vi "ixon.vi"() -> ()   [LabVIEW 2016]
uses:
  <userlib>/atmcd64d.llb/Shutter_mode typedef.ctl
  <userlib>/atmcd64d.llb/Error Code Enum typedef.ctl
  <userlib>/atmcd64d.llb/Shutter_type typedef.ctl
  <userlib>/atmcd64d.llb/FanMode_mode typedef.ctl
  <userlib>/atmcd64d.llb/ReadMode_mode typedef.ctl
  <userlib>/atmcd64d.llb/HSSpeed_type typedef.ctl
  <userlib>/atmcd64d.llb/AcquisitionMode_mode typedef.ctl
  <vilib>/Utility/miscctls.llb/LVStringsAndValuesArrayTypeDef_U16.ctl
  <vilib>/Instr/_visa.llb/VISA Configure Serial Port (Instr).vi
panel:
  in  "Tab Control":T1(tab)
  out "DLL error code from ini":u32
  out "model":string
  out "temp. status 2":T2
  out "temperature 2":i32
  in  "set temperature 2":i32
  in  "VSS (s)":u16(ring) items=["0.300000", "0.500000", "0.900000", "1.700000", "3.300000"]
  in  "HSS (MHz)":i32(ring) items=["3", "1"]
  in  "shutter":T3
  in  "exposure time (s)":sgl=0.01 step=0.001 format="%.4f"
  in  "Take shot":bool
  out "aquire status":T2
  out "Return  from Get Acquired Data":u32
  in  "live view":bool
  in  "capture stop":bool
  out "Allowed \nVertical \nShift Speed\n(seconds)":sgl[](array[numeric])
  out "Allowed \nHorizontal \nShift Speed\n(MHz)":sgl[](array[numeric])
  in  "File name":string
  in  "Path":path=path "C:/Users/Administrator/Desktop/test.tiff"
  in  "scan":bool
  in  "total scan length(mm)":dbl=25.0
  in  "distance(mm)":i32=153
  in  "lens focal length(mm)":i32=23
  out "recovering temperature":bool
  in  "Bandwidth":dbl
  in  "scan again":bool
  out "Waveform Graph":i32[](graph)
  in  "index (page) 2":i32(slide)=200 scale=0.0..512.0
  in  "Y Scale Range (mm)":dbl=67.0
  in  "stop":bool
  in  "file path (use dialog)":path=path "C:/Users/Administrator/Desktop/binary.txt"
  out "size(s) 2":i32[](array[numeric])
  out "size(s)":i32[](array[numeric])
  out "Numeric 2":i32
  out "status":T2
  out "Return  from Get Acquired Data 2":u32
  out "Intensity Graph 2":i32[][](graph)
  out "DLL error code":u32
  out "Intensity Graph":i32[][](graph)
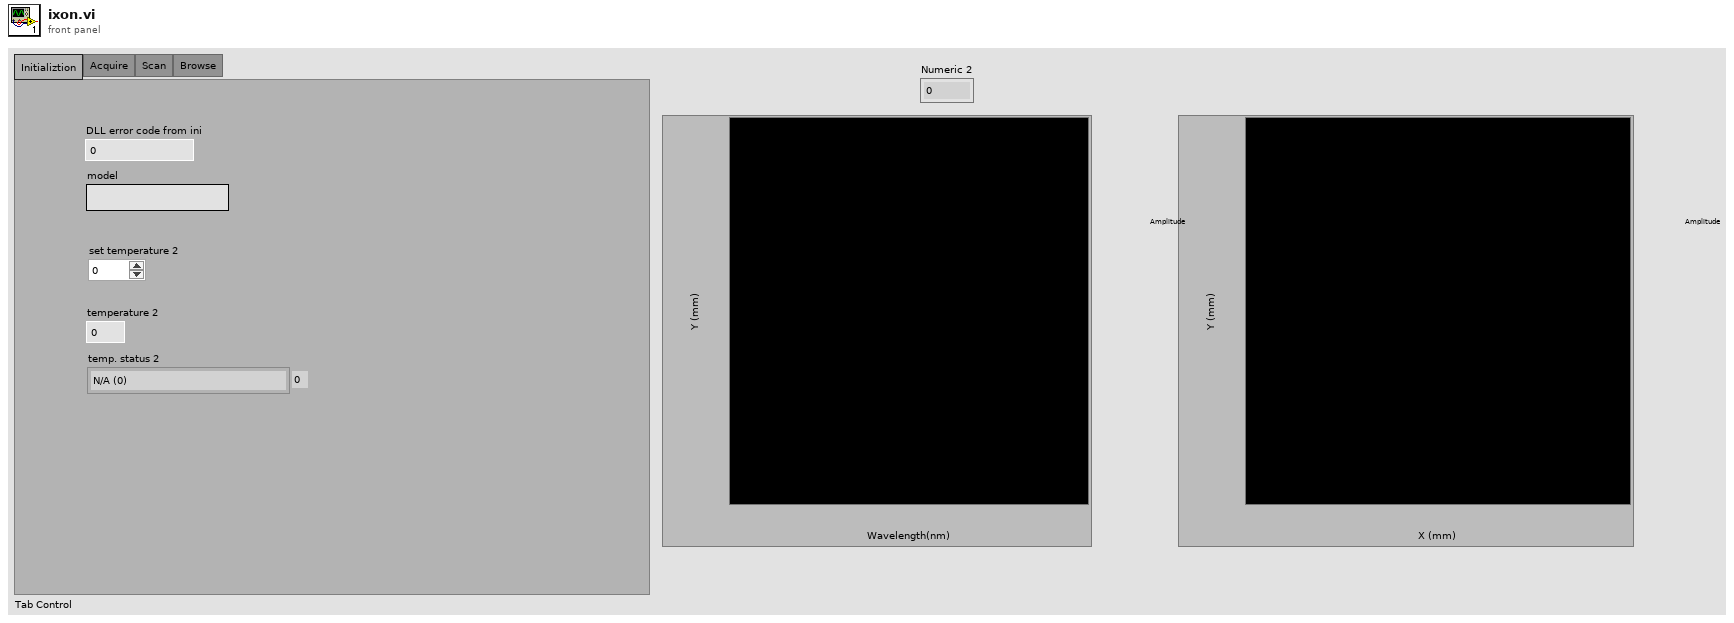
[diagram p1: front panel]
types:
  T1 = enum32{"Initializtion", "Acquire", "Scan", "Browse"}
  T2 = typedef "Error Code Enum typedef.ctl" = enum32{"N/A (0)", "DRV_ERROR_CODES", "DRV_SUCCESS", "DRV_VXDNOTINSTALLED", "DRV_ERROR_SCAN", "DRV_ERROR_CHECK_SUM", "DRV_ERROR_FILELOAD", "DRV_UNKNOWN_FUNC", "DRV_ERROR_VXD_INIT", "DRV_ERROR_ADDRESS", "DRV_ERROR_PAGELOCK", "DRV_ERROR_PAGEUNLOCK", "DRV_ERROR_BOARDTEST", "DRV_ERROR_ACK", "DRV_ERROR_UP_FIFO", "DRV_ERROR_PATTERN", "N/A (16)", "DRV_ACQUISITION_ERRORS", "DRV_ACQ_BUFFER", "DRV_ACQ_DOWNFIFO_FULL", "DRV_PROC_UNKONWN_INSTRUCTION", "DRV_ILLEGAL_OP_CODE", "DRV_KINETIC_TIME_NOT_MET", "DRV_ACCUM_TIME_NOT_MET", "DRV_NO_NEW_DATA", "N/A (25)", "DRV_SPOOLERROR", "N/A (27)", "N/A (28)", "N/A (29)", "N/A (30)", "N/A (31)", "N/A (32)", "DRV_TEMPERATURE_CODES", "DRV_TEMPERATURE_OFF", "DRV_TEMPERATURE_NOT_STABILIZED", "DRV_TEMPERATURE_STABILIZED", "DRV_TEMPERATURE_NOT_REACHED", "DRV_TEMPERATURE_OUT_RANGE", "DRV_TEMPERATURE_NOT_SUPPORTED", "DRV_TEMPERATURE_DRIFT", "N/A (41)", "N/A (42)", "N/A (43)", "N/A (44)", "N/A (45)", "N/A (46)", "N/A (47)", "N/A (48)", "DRV_GENERAL_ERRORS", "DRV_INVALID_AUX", "DRV_COF_NOTLOADED", "DRV_FPGAPROG", "DRV_FLEXERROR", "DRV_GPIBERROR", "N/A (55)", "N/A (56)", "N/A (57)", "N/A (58)", "N/A (59)", "N/A (60)", "N/A (61)", "N/A (62)", "N/A (63)", "DRV_DATATYPE", "DRV_DRIVER_ERRORS", "DRV_P1INVALID", "DRV_P2INVALID", "DRV_P3INVALID", "DRV_P4INVALID", "DRV_INIERROR", "DRV_COFERROR", "DRV_ACQUIRING", "DRV_IDLE", "DRV_TEMPCYCLE", "DRV_NOT_INITIALIZED", "DRV_P5INVALID", "DRV_P6INVALID", "DRV_INVALID_MODE", "DRV_INVALID_FILTER", "DRV_I2CERRORS", "DRV_I2CDEVNOTFOUND", "DRV_I2CTIMEOUT", "DRV_P7INVALID", "N/A (84)", "N/A (85)", "N/A (86)", "N/A (87)", "N/A (88)", "N/A (89)", "DRV_IOCERROR", "DRV_VRMVERSIONERROR"}
  T3 = typedef "Shutter_mode typedef.ctl" = enum16{"Auto", "Open", "Close", "N/A (3)", "Open FVB Series", "Open Any Series"}
  T4 = typedef "FanMode_mode typedef.ctl" = enum16{"fan on full", "fan on low", "fan off"}
  T5 = typedef "Shutter_type typedef.ctl" = enum16{"TTL Low", "TTL High"}
  T6 = typedef "LVStringsAndValuesArrayTypeDef_U16.ctl" = cluster{"String":string, "Value":u16}[]
  T7 = typedef "AcquisitionMode_mode typedef.ctl" = enum16{"Reserved (0)", "Single Scan", "Accumulate", "Kinetics", "Fast Kinetics", "Run Till Abort", "Reserved (6)", "Reserved (7)", "Reserved (8)", "Time Delayed Integration"}
  T8 = typedef "ReadMode_mode typedef.ctl" = enum16{"Full Vertical Binning", "Multi-Track", "Random-Track", "Single-Track", "Image"}
  T9 = typedef "HSSpeed_type typedef.ctl" = enum16{"EM Amp", "Conventional Amp"}
  T10 = enum16{"big-endian, network order", "native, host order", "little-endian"}
  T11 = typedef "LVPoint32TypeDef.ctl" = cluster{"Horizontal":i32, "Vertical":i32}
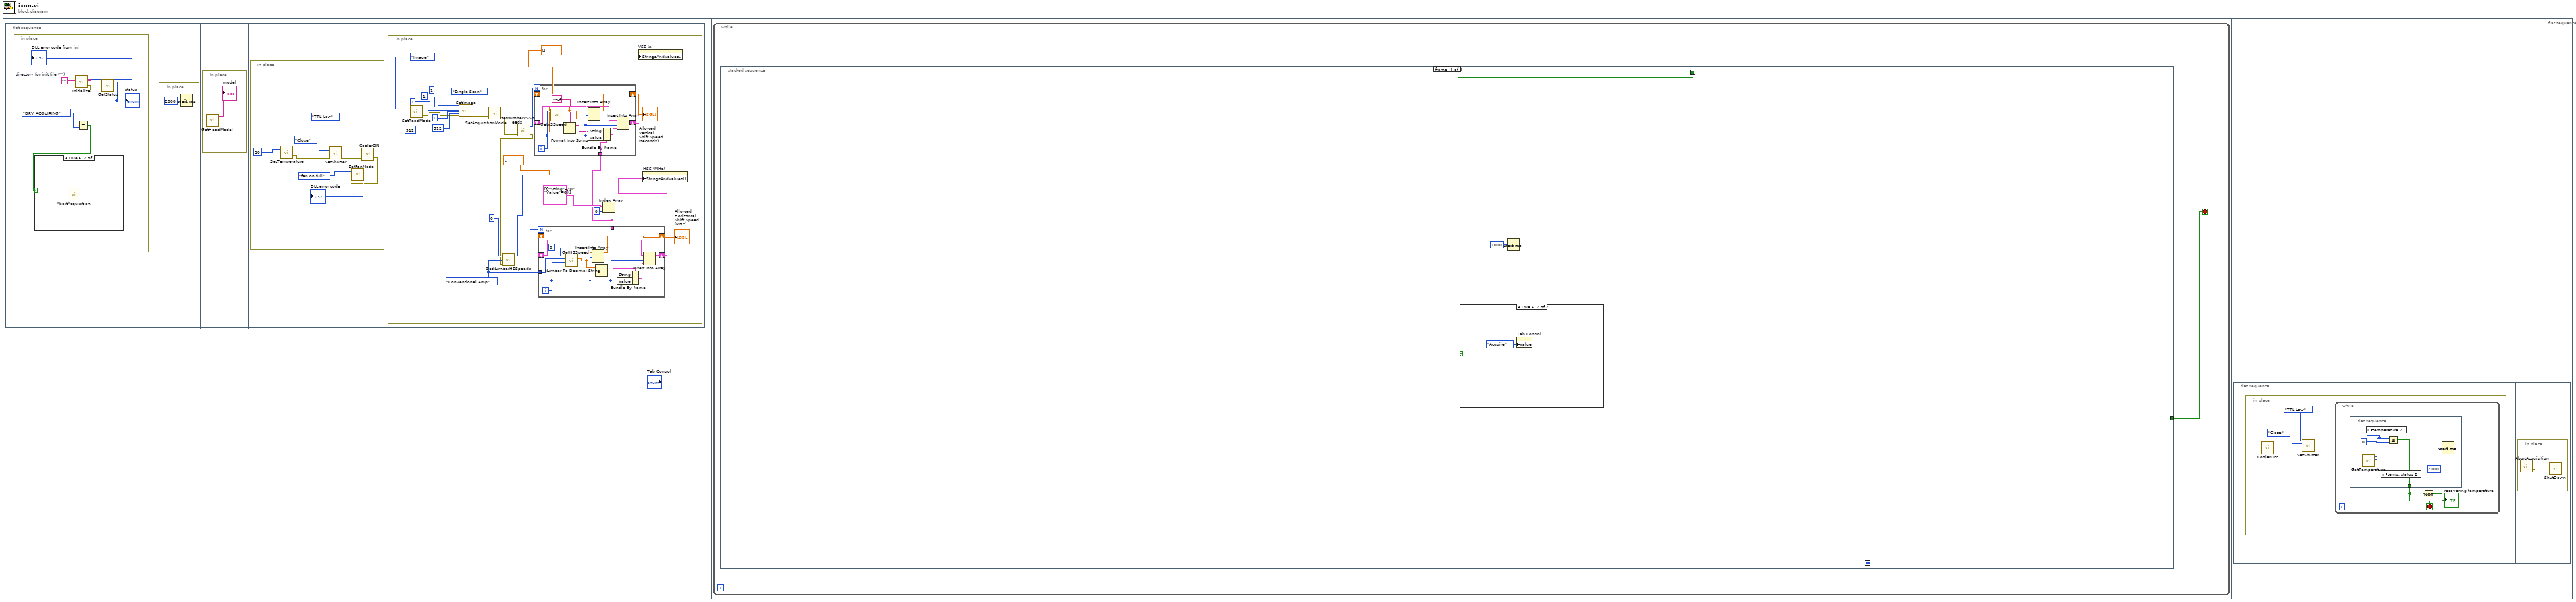
[diagram p0: block diagram]
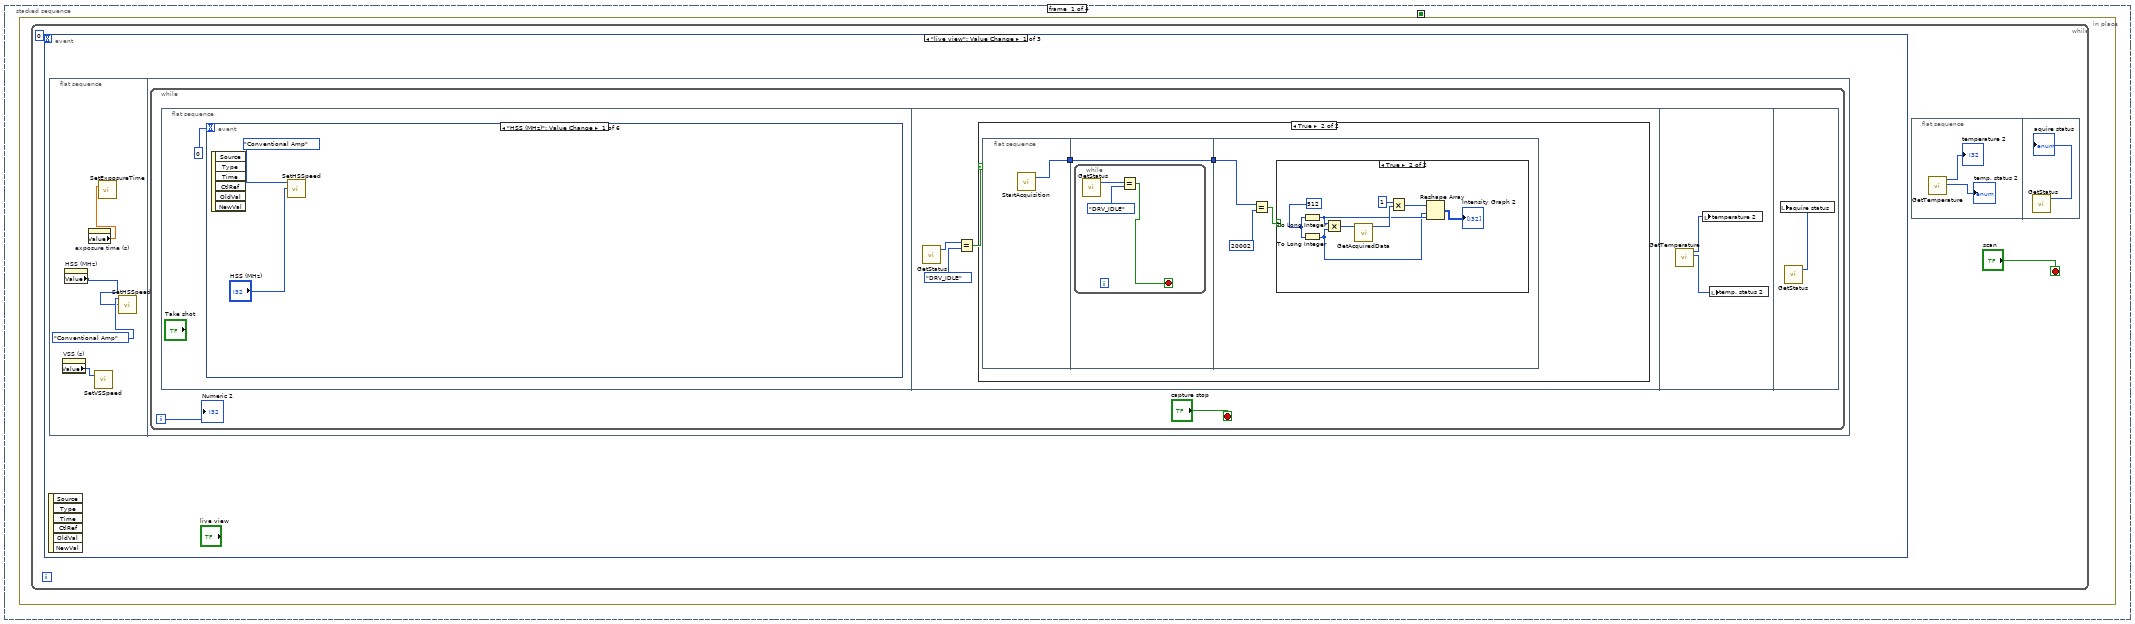
[diagram p3: hidden frame]
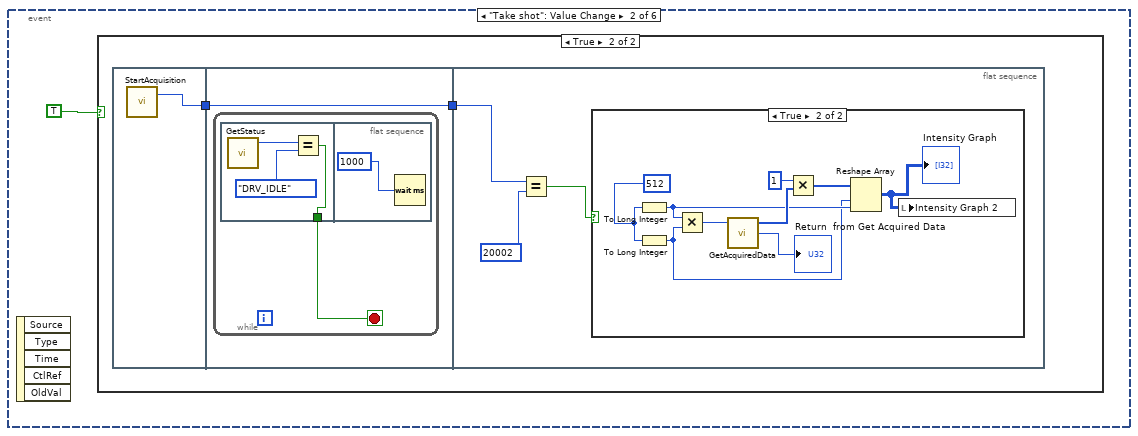
[diagram p4: hidden frame]
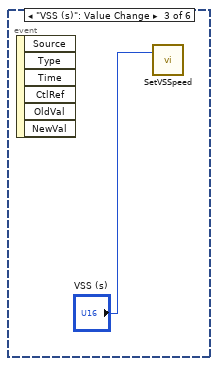
[diagram p7: hidden frame]
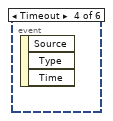
[diagram p8: hidden frame]
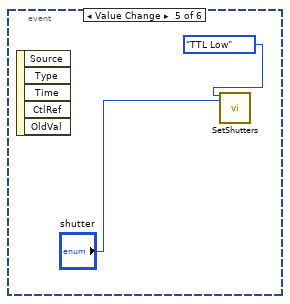
[diagram p9: hidden frame]
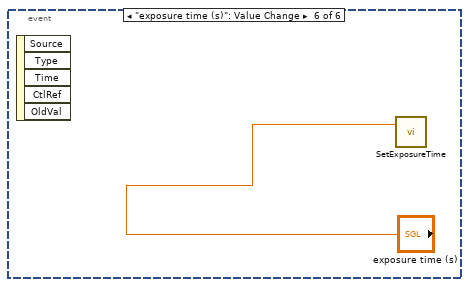
[diagram p10: hidden frame]
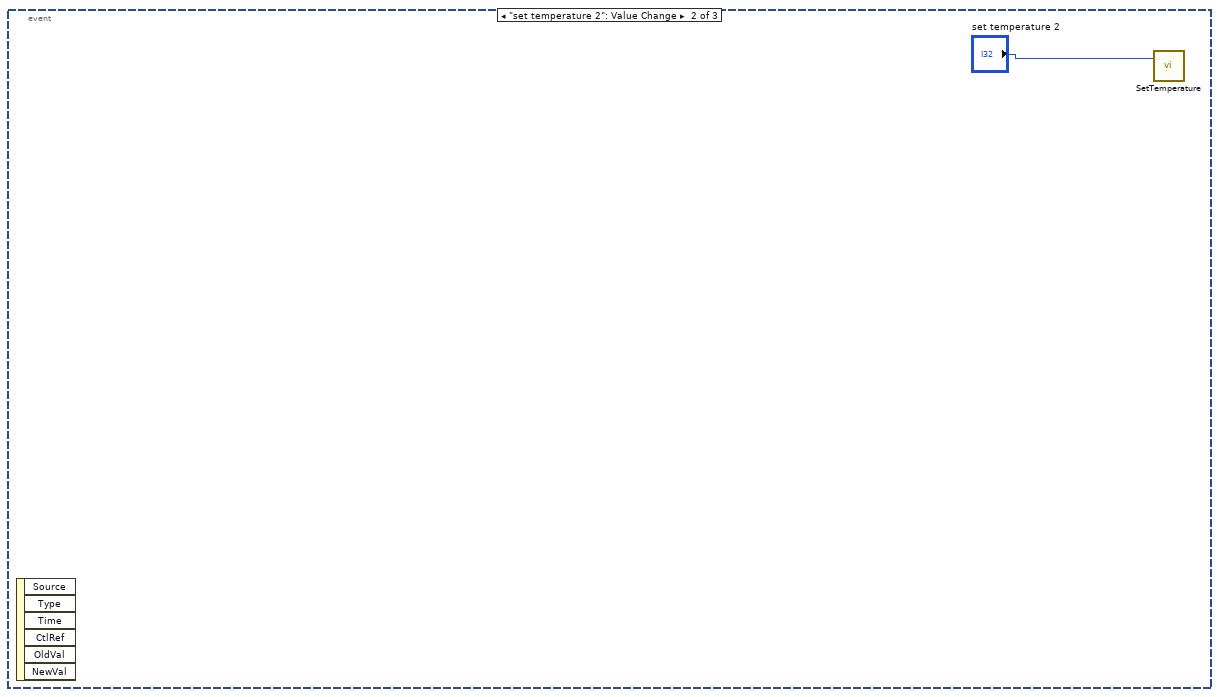
[diagram p13: hidden frame]
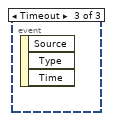
[diagram p14: hidden frame]
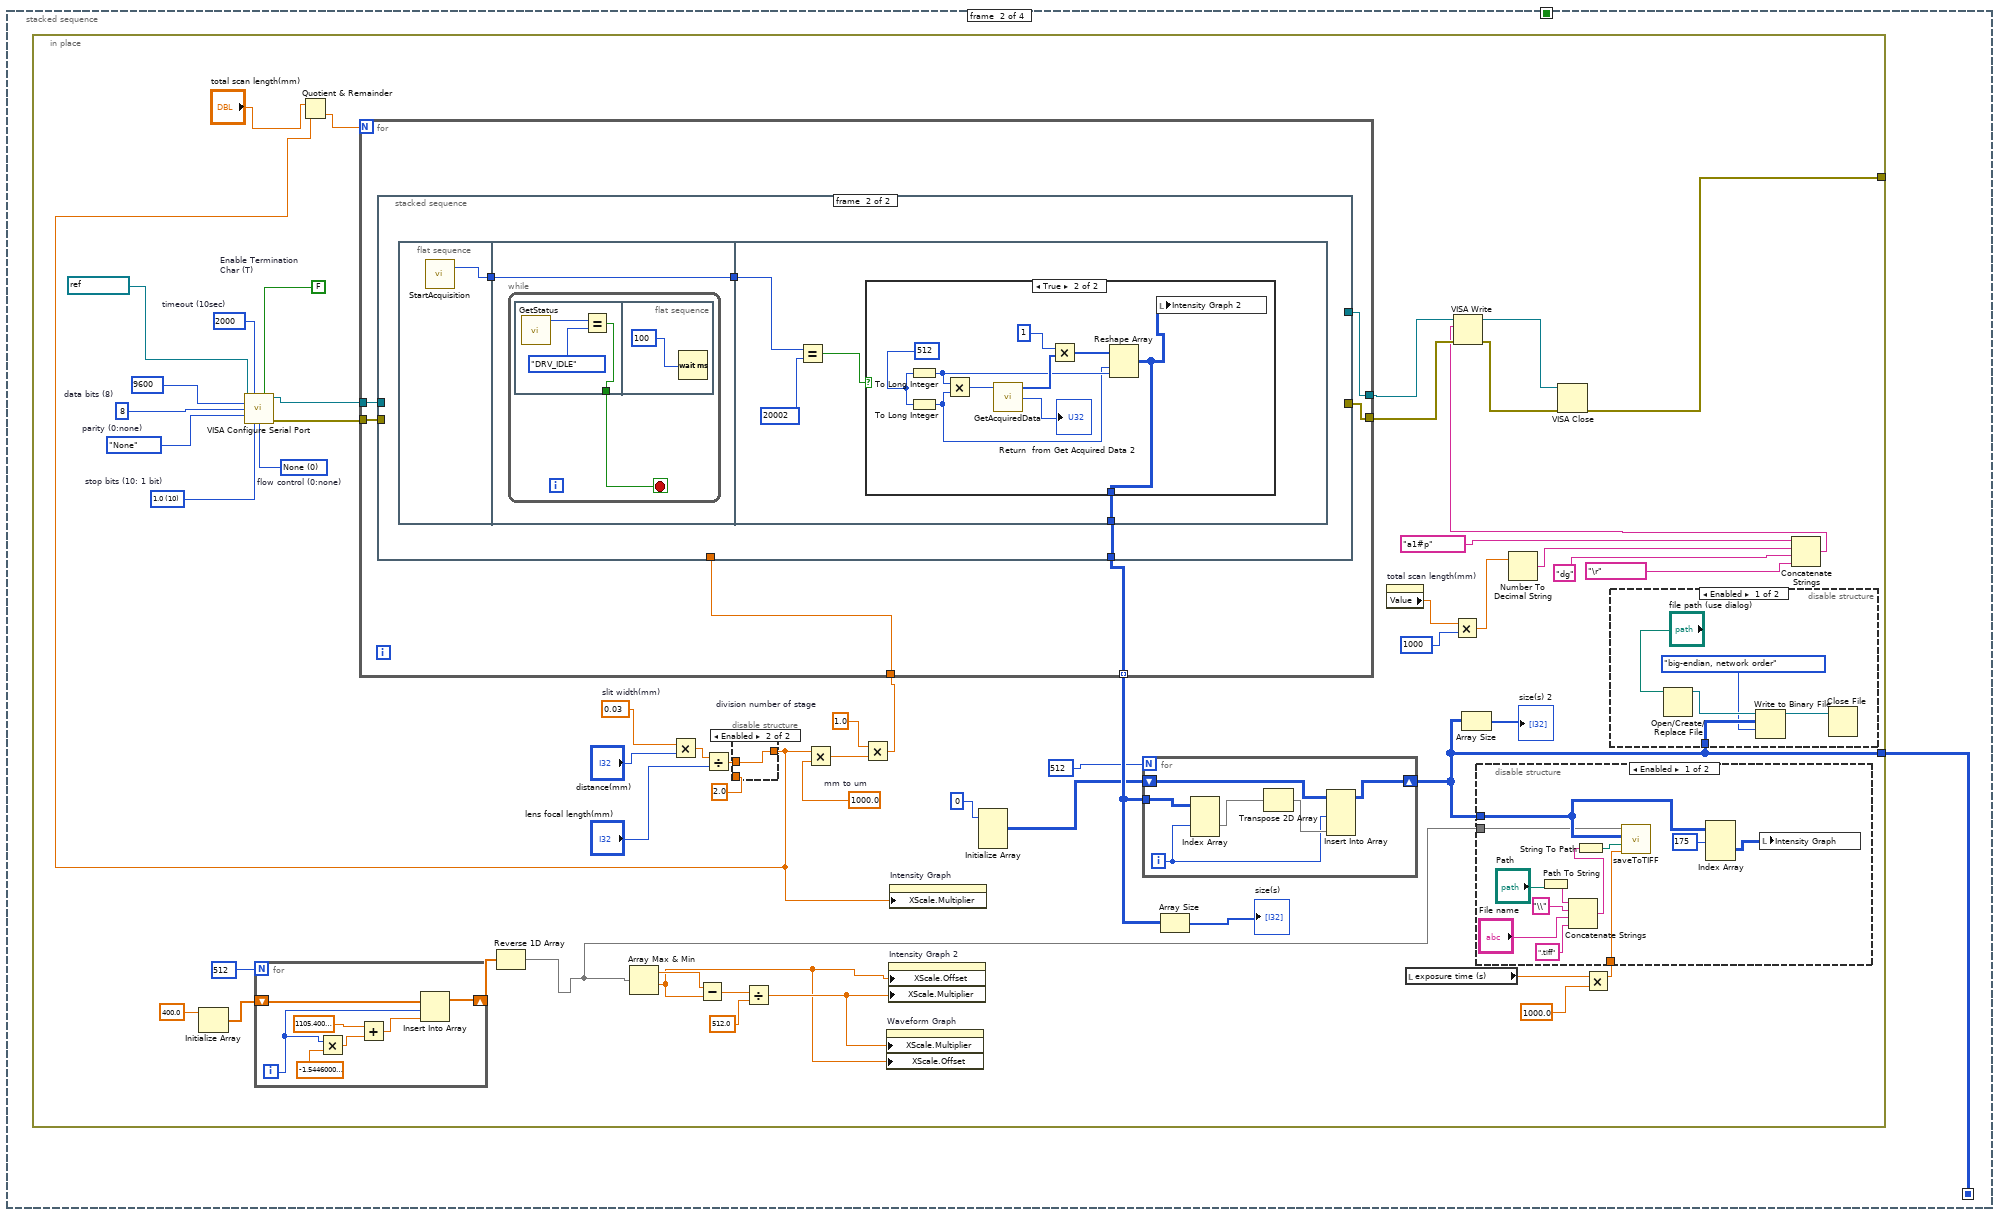
[diagram p15: hidden frame]
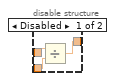
[diagram p17: hidden frame]
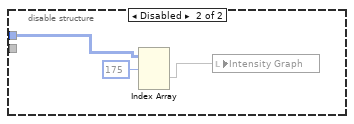
[diagram p18: hidden frame]
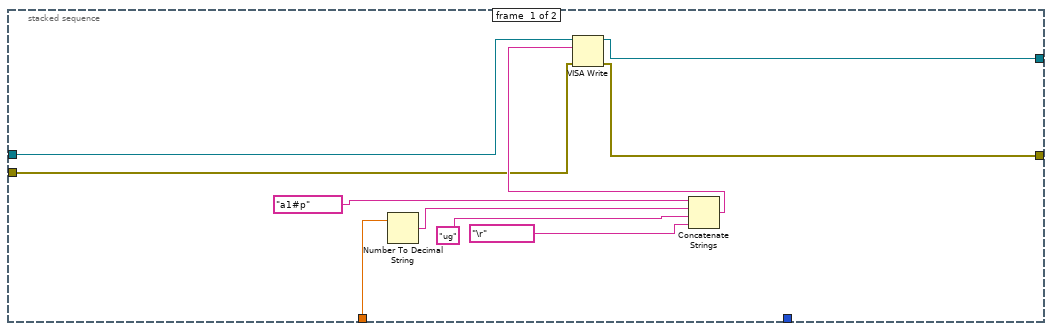
[diagram p19: hidden frame]
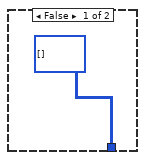
[diagram p20: hidden frame]
diagram:
  n1 = flat-sequence {
    frame #0 {
      n2 = flat-sequence {
        frame #0 {
          n3 = in-place {
            w6 = ""  # directory for init file ("")
            n4 = call <userlib>:"Initialize.vi"("directory (\"\")"=w6) -> ("error out"=w4:errorcluster, "DLL error code"=→"DLL error code from ini":u32)  [unwired: 1 in]
            n5 = call <userlib>:"GetStatus.vi"("error in (no error)"=w4) -> ("status"=w3:T2)  [unwired: 2 in, 2 out]
            "status" <- w3
            n6 = Equal?(x=w3, y=Error_Code_Enum_typedef."DRV_ACQUIRING" ("status")) -> (x = y?=w1:bool)
            n7 = case shown="True" w1 {
              frame False {
              }
              frame True {
                n8 = call <userlib>:"AbortAcquisition.vi"() -> ()  [unwired: 2 in, 2 out]
              }
            }
          }
        }
        frame #1 {
          n9 = in-place {
            n10 = Wait (ms)(milliseconds to wait=u32 2000) -> ()  [unwired: 1 out]
          }
        }
        frame #2 {
          n11 = in-place {
            n12 = call <userlib>:"GetHeadModel.vi"() -> ("model"=→"model":string)  [unwired: 3 in, 2 out]
          }
        }
        frame #3 {
          n13 = in-place {
            n14 = call <userlib>:"SetTemperature.vi"("temperature"=20) -> ("error out"=w12:errorcluster)  [unwired: 1 in, 1 out]
            n15 = call <userlib>:"SetShutter.vi"("type"=Shutter_type_typedef."TTL Low", "mode"=Shutter_mode_typedef."Close", "error in (no error)"=w12) -> ("error out"=w13:errorcluster)  [unwired: 11 in, 1 out]
            n16 = call <userlib>:"CoolerON.vi"("error in (no error)"=w13) -> ("error out"=w10:errorcluster)  [unwired: 1 in, 1 out]
            n17 = call <userlib>:"SetFanMode.vi"("error in (no error)"=w10, "mode"=FanMode_mode_typedef."fan on full") -> ("DLL error code"=→"DLL error code":u32)  [unwired: 1 out]
          }
        }
        frame #4 {
          n18 = in-place {
            w29 = HSSpeed_type_typedef."Conventional Amp" ("type")
            n19 = call <userlib>:"SetReadMode.vi"("mode"=ReadMode_mode_typedef."Image") -> ("error out"=w34:errorcluster)  [unwired: 1 in, 1 out]
            n20 = call <userlib>:"SetImage.vi"("hbin"=1, "vbin"=1, "hstart"=1, "hend"=512, "vstart"=1, "vend"=512, "error in (no error)"=w34) -> ("error out"=w24:errorcluster)  [unwired: 19 in, 1 out]
            n21 = call <userlib>:"SetAcquisitionMode.vi"("error in (no error)"=w24, "mode"=AcquisitionMode_mode_typedef."Single Scan") -> ("error out"=w23:errorcluster)  [unwired: 1 out]
            n22 = call <userlib>:"GetNumberVSSpeeds.vi"("error in (no error)"=w23) -> ("error out"=w25:errorcluster, "number"=w32:i32)  [unwired: 2 in, 1 out]
            n23 = call <userlib>:"GetNumberHSSpeeds.vi"("error in (no error)"=w25, "type"=w29, "channel"=0) -> ("number"=w28:i32)  [unwired: 2 out]
            n24 = Index Array(array=T6 [{"String"="0", "Value"=0}] ("Strings And Values []"), index=0) -> (element=w18:cluster{"String":string, "Value":u16})
            n25 = for {
              N: w32 -> [_]
              shift-right: [w61] -> w33
              shift-left: sgl[] [] -> [w62]
              tunnel: w18 -> [w60]
              shift-right: [w57] -> w17
              shift-left: _ -> [w56]
              i -> [w58]
              n26 = call <userlib>:"GetVSSpeed.vi"("index"=w58) -> ("speed"=w54:sgl)  [unwired: 2 in, 2 out]
              n27 = Format Into String(format string="%f", w54) -> (resulting string=w55:string)  [unwired: 2 in, 1 out]
              n28 = Insert Into Array(array=w62, index=w58, new element=w54) -> (w61:sgl[])
              n29 = Bundle By Name(cluster=w60, "String"=w55, "Value"=w58) -> (w59:cluster{"String":string, "Value":u16})
              n30 = Insert Into Array(array=w56, index=w58, new element=w59) -> (w57:cluster{"String":string, "Value":u16}[])
            }
            "Allowed \nVertical \nShift Speed\n(seconds)" <- w33
            n31 = for {
              N: w28 -> [_]
              tunnel: w29 -> [w51]
              shift-right: [w49] -> w26
              shift-left: sgl[] [] -> [w50]
              shift-right: [w44] -> w21
              shift-left: _ -> [w43]
              tunnel: w18 -> [w42]
              i -> [w45]
              n32 = call <userlib>:"GetHSSpeed.vi"("index"=w45, "type"=w51, "channel"=0) -> ("speed"=w48:sgl)  [unwired: 2 in, 2 out]
              n33 = Insert Into Array(array=w50, index=w45, new element=w48) -> (w49:sgl[])
              n34 = Number To Decimal String(number=w48) -> (decimal integer string=w47:string)  [unwired: 1 in]
              n35 = Bundle By Name(cluster=w42, "String"=w47, "Value"=w45) -> (w46:cluster{"String":string, "Value":u16})
              n36 = Insert Into Array(array=w43, index=w45, new element=w46) -> (w44:cluster{"String":string, "Value":u16}[])
            }
            "Allowed \nHorizontal \nShift Speed\n(MHz)" <- w26
            n37 = property on="VSS (s)" class="Ring (strict)"("StringsAndValues[]"=w17) -> ()  [unwired: 2 in, 2 out]
            n38 = property on="HSS (MHz)" class="Ring (strict)"("StringsAndValues[]"=w21) -> ()  [unwired: 2 in, 2 out]
          }
        }
      }
    }
    frame #1 {
      n39 = while {
        stop <- w63 stop-if-true
        n40 = stacked-sequence {
          seq-local: [_ w129 _ _] -> [_ _ w265 _]
          seq-local: [_ _ w263 _] -> [_ _ _ w364]
          tunnel: [_ _ w264 _] -> w63
          frame #0 {
            n41 = in-place {
              n42 = while {
                stop <- "scan" stop-if-true
                n43 = event shown="[0] \"live view\": Value Change" {
                  selector: _ -> [_ _ _]
                  dyn-events: _ -> [_ _ _]
                  timeout: 0 -> [_ _ _]
                  event "live view": Value Change {
                    n44 = event-data() -> ()  [unwired: 1 in, 6 out]
                    n45 = flat-sequence {
                      frame #0 {
                        n46 = property on="VSS (s)" class="Ring (strict)"() -> ("Value"=w67:u16)  [unwired: 2 in, 2 out]
                        n47 = property on="HSS (MHz)" class="Ring (strict)"() -> ("Value"=w66:i32)  [unwired: 2 in, 2 out]
                        n48 = property on="exposure time (s)" class="DigNum (strict)"() -> ("Value"=w69:sgl)  [unwired: 2 in, 2 out]
                        n49 = call <userlib>:"SetVSSpeed.vi"("index"=w67) -> ()  [unwired: 1 in, 2 out]
                        n50 = call <userlib>:"SetExposureTime.vi"("time"=w69) -> ()  [unwired: 1 in, 2 out]
                        n51 = call <userlib>:"SetHSSpeed.vi"("index"=w66, "type"=HSSpeed_type_typedef."Conventional Amp") -> ()  [unwired: 2 in, 2 out]
                      }
                      frame #1 {
                        n52 = while {
                          i -> [w70]
                          stop <- "capture stop" stop-if-true
                          n53 = flat-sequence {
                            frame #0 {
                              n54 = event shown="[0] \"HSS (MHz)\": Value Change" {
                                selector: _ -> [_ _ _ _ _ _]
                                dyn-events: _ -> [_ _ _ _ _ _]
                                timeout: 0 -> [_ _ _ _ _ _]
                                event "HSS (MHz)": Value Change {
                                n55 = event-data() -> ()  [unwired: 1 in, 6 out]
                                n56 = call <userlib>:"SetHSSpeed.vi"("index"="HSS (MHz)", "type"=HSSpeed_type_typedef."Conventional Amp") -> ()  [unwired: 2 in, 2 out]
                                }
                                event "Take shot": Value Change {
                                n57 = event-data() -> ()  [unwired: 1 in, 5 out]
                                n58 = case shown="True" TRUE {
                                frame False {
                                }
                                frame True {
                                n59 = flat-sequence {
                                tunnel: [w78] -> w77
                                tunnel: w77 -> [w79]
                                tunnel: [w79] -> w76
                                tunnel: w76 -> [w87]
                                frame #0 {
                                n60 = call <userlib>:"StartAcquisition.vi"() -> ("DLL error code"=w78:u32)  [unwired: 2 in, 1 out]
                                }
                                frame #1 {
                                n61 = while {
                                stop <- w80 stop-if-true
                                n62 = flat-sequence {
                                tunnel: [w81] -> w80
                                frame #0 {
                                n63 = call <userlib>:"GetStatus.vi"() -> ("status"=w82:T2)  [unwired: 3 in, 2 out]
                                n64 = Equal?(x=w82, y=Error_Code_Enum_typedef."DRV_IDLE" ("status")) -> (x = y?=w81:bool)
                                }
                                frame #1 {
                                n65 = Wait (ms)(milliseconds to wait=u32 1000) -> ()  [unwired: 1 out]
                                }
                                }
                                }
                                }
                                frame #2 {
                                n66 = Equal?(x=w87, y=u32 20002) -> (x = y?=w85:bool)
                                n67 = case shown="True" w85 {
                                frame False {
                                }
                                frame True {
                                w89 = 512
                                n68 = To Long Integer(number=w89) -> (32bit integer=w91:i32)
                                n69 = To Long Integer(number=w89) -> (32bit integer=w90:i32)
                                n70 = Multiply(x=w91, y=w90) -> (x*y=w95:i32)
                                n71 = call <userlib>:"GetAcquiredData.vi"("size"=w95) -> ("DLL error code"=→"Return  from Get Acquired Data":u32, "array"=w93:i32[])  [unwired: 2 in, 1 out]
                                n72 = Multiply(x=1, y=w93) -> (x*y=w92:i32[])
                                n73 = Reshape Array(w92, w90, w91) -> (w88:i32[][])
                                "Intensity Graph" <- w88
                                n74 = local write "Intensity Graph 2"(w88) -> ()
                                }
                                }
                                }
                                }
                                }
                                }
                                }
                                event "VSS (s)": Value Change {
                                n75 = event-data() -> ()  [unwired: 1 in, 6 out]
                                n76 = call <userlib>:"SetVSSpeed.vi"("index"="VSS (s)") -> ()  [unwired: 1 in, 2 out]
                                }
                                event Timeout {
                                n77 = event-data() -> ()  [unwired: 1 in, 3 out]
                                }
                                event Value Change {
                                n78 = event-data() -> ()  [unwired: 1 in, 5 out]
                                n79 = call <userlib>:"SetShutters.vi"("type"=Shutter_type_typedef."TTL Low", "mode"="shutter") -> ()  [unwired: 16 in, 2 out]
                                }
                                event "exposure time (s)": Value Change {
                                n80 = event-data() -> ()  [unwired: 1 in, 5 out]
                                n81 = call <userlib>:"SetExposureTime.vi"("time"="exposure time (s)") -> ()  [unwired: 1 in, 2 out]
                                }
                              }
                            }
                            frame #1 {
                              n82 = call <userlib>:"GetStatus.vi"() -> ("status"=w103:T2)  [unwired: 3 in, 2 out]
                              n83 = Equal?(x=w103, y=Error_Code_Enum_typedef."DRV_IDLE" ("status")) -> (x = y?=w101:bool)
                              n84 = case shown="True" w101 {
                                frame False {
                                }
                                frame True {
                                n85 = flat-sequence {
                                tunnel: [w106] -> w105
                                tunnel: w105 -> [w107]
                                tunnel: [w107] -> w104
                                tunnel: w104 -> [w113]
                                frame #0 {
                                n86 = call <userlib>:"StartAcquisition.vi"() -> ("DLL error code"=w106:u32)  [unwired: 2 in, 1 out]
                                }
                                frame #1 {
                                n87 = while {
                                stop <- w110 stop-if-true
                                n88 = call <userlib>:"GetStatus.vi"() -> ("status"=w108:T2)  [unwired: 3 in, 2 out]
                                n89 = Equal?(x=w108, y=Error_Code_Enum_typedef."DRV_IDLE" ("status")) -> (x = y?=w110:bool)
                                }
                                }
                                frame #2 {
                                n90 = Equal?(x=w113, y=u32 20002) -> (x = y?=w111:bool)
                                n91 = case shown="True" w111 {
                                frame False {
                                }
                                frame True {
                                w115 = 512
                                n92 = To Long Integer(number=w115) -> (32bit integer=w117:i32)
                                n93 = To Long Integer(number=w115) -> (32bit integer=w116:i32)
                                n94 = Multiply(x=w117, y=w116) -> (x*y=w121:i32)
                                n95 = call <userlib>:"GetAcquiredData.vi"("size"=w121) -> ("array"=w119:i32[])  [unwired: 2 in, 2 out]
                                n96 = Multiply(x=1, y=w119) -> (x*y=w118:i32[])
                                n97 = Reshape Array(w118, w116, w117) -> (→"Intensity Graph 2":i32[][])
                                }
                                }
                                }
                                }
                                }
                              }
                            }
                            frame #2 {
                              n98 = call <userlib>:"GetTemperature.vi"() -> ("status"=w122:T2, "temperature"=w123:i32)  [unwired: 4 in, 2 out]
                              n99 = local write "temperature 2"(w123) -> ()
                              n100 = local write "temp. status 2"(w122) -> ()
                            }
                            frame #3 {
                              n101 = call <userlib>:"GetStatus.vi"() -> ("status"=w124:T2)  [unwired: 3 in, 2 out]
                              n102 = local write "aquire status"(w124) -> ()
                            }
                          }
                          "Numeric 2" <- w70
                        }
                      }
                    }
                  }
                  event "set temperature 2": Value Change {
                    n103 = event-data() -> ()  [unwired: 1 in, 6 out]
                    n104 = call <userlib>:"SetTemperature.vi"("temperature"="set temperature 2") -> ()  [unwired: 1 in, 2 out]
                  }
                  event Timeout {
                    n105 = event-data() -> ()  [unwired: 1 in, 3 out]
                  }
                }
                n106 = flat-sequence {
                  frame #0 {
                    n107 = call <userlib>:"GetTemperature.vi"() -> ("status"=→"temp. status 2":T2, "temperature"=→"temperature 2":i32)  [unwired: 4 in, 2 out]
                  }
                  frame #1 {
                    n108 = call <userlib>:"GetStatus.vi"() -> ("status"=→"aquire status":T2)  [unwired: 3 in, 2 out]
                  }
                }
              }
            }
          }
          frame #1 {
            n109 = in-place {
              in-place-border: [w148] -> _
              in-place-border: [w147] -> w129
              w169 = 1.0  # division number of stage
              w171 = 1000.0  # mm to um
              w175 = 0.03  # slit width(mm)
              w179 = u16 0 items=["None", "XON/XOFF", "RTS/CTS", "XON/XOFF & RTS/CTS", "DTR/DSR", "XON/XOFF & DTR/DSR"]  # flow control (0:none)
              w180 = u16 10 items=["1.0"=10, "1.5"=15, "2.0"=20]  # stop bits (10: 1 bit)
              w181 = FALSE  # Enable Termination Char (T)
              w182 = u32 2000  # timeout (10sec)
              w183 = enum16{"None", "Odd", "Even", "Mark", "Space"}."None"  # parity (0:none)
              w184 = u16 8  # data bits (8)
              n110 = Initialize Array(sgl 400.0 ("element")) -> (w141:sgl[])  [unwired: 1 in]
              n111 = call-poly "VISA Configure Serial Port"("VISA resource name"=refnum<visa-resource-name> "COM4", "timeout (10sec)"=w182, "Enable Termination\nChar (T)"=w181, "baud rate (9600)"=u32 9600, "data bits (8)"=w184, "parity (0:none)"=w183, "stop bits (10: 1 bit)"=w180, "flow control (0:none)"=w179) -> ("VISA resource name out"=w177:refnum<visa-resource-name>, "error out"=w176:errorcluster)  [unwired: 6 in]
              n112 = for {
                N: 512 -> [_]
                shift-right: [w261] -> w142
                shift-left: w141 -> [w262]
                i -> [w260]
                n113 = Multiply(x=w260, y=sgl -1.5446) -> (x*y=w258:sgl)
                n114 = Add(x=sgl 1105.4, y=w258) -> (x+y=w256:sgl)
                n115 = Insert Into Array(array=w262, index=w260, new element=w256) -> (w261:sgl[])
              }
              n116 = Reverse 1D Array(array=w142) -> (reversed array=w133:sgl[])
              n117 = Array Max & Min(array=w133) -> (max value=w143:sgl, min value=w137:sgl)  [unwired: 2 out]
              n118 = Multiply(x=w175, y="distance(mm)") -> (x*y=w173:dbl)
              n119 = Subtract(x=w143, y=w137) -> (x-y=w144:sgl)
              n120 = Divide(x=w173, y="lens focal length(mm)") -> (x/y=w150:dbl)
              n121 = disable-structure shown="Enabled" {
                disable-tunnel: w150 -> [w193 w194]
                disable-tunnel: 2.0 ("y") -> [w192 _]
                disable-tunnel: [w191 w194] -> w131
                frame Disabled {
                  n122 = Divide(x=w193, y=w192) -> (x/y=w191:dbl)
                }
                frame Enabled {
                }
              }
              n123 = Quotient & Remainder(x="total scan length(mm)", y=w131) -> (floor(x/y)=w130:dbl)  [unwired: 1 out]
              n124 = Divide(x=w144, y=sgl 512.0) -> (x/y=w138:sgl)
              n125 = Multiply(x=w131, y=w171) -> (x*y=w170:dbl)
              n126 = Multiply(x=w169, y=w170) -> (x*y=w146:dbl)
              n127 = for {
                N: w130 -> [_]
                tunnel: w177 -> [w221]
                tunnel: w176 -> [w220]
                tunnel: [w217] -> w168
                tunnel: [w216] -> w167
                tunnel: [w219] -> w158 mode=indexing
                tunnel: w146 -> [w218]
                n128 = stacked-sequence {
                  tunnel: w221 -> [w230 _]
                  tunnel: w220 -> [w229 _]
                  tunnel: [w223 _] -> w217
                  tunnel: [_ w232] -> w219
                  tunnel: w218 -> [w224 _]
                  tunnel: [w222 _] -> w216
                  frame #0 {
                    n129 = Number To Decimal String(number=w224) -> (decimal integer string=w225:string)  [unwired: 1 in]
                    n130 = Concatenate Strings("a1#p" ("string"), w225, "ug" ("string"), "\r" ("write buffer")) -> (w231:string)
                    n131 = VISA Write(VISA resource name=w230, write buffer=w231, error in (no error)=w229) -> (VISA resource name out=w223:refnum<visa-resource-name>, error out=w222:errorcluster)  [unwired: 1 out]
                  }
                  frame #1 {
                    n132 = flat-sequence {
                      tunnel: [w235] -> w234
                      tunnel: w234 -> [w236]
                      tunnel: [w236] -> w233
                      tunnel: w233 -> [w245]
                      tunnel: [w242] -> w232
                      frame #0 {
                        n133 = call <userlib>:"StartAcquisition.vi"() -> ("DLL error code"=w235:u32)  [unwired: 2 in, 1 out]
                      }
                      frame #1 {
                        n134 = while {
                          stop <- w237 stop-if-true
                          n135 = flat-sequence {
                            tunnel: [w238] -> w237
                            frame #0 {
                              n136 = call <userlib>:"GetStatus.vi"() -> ("status"=w239:T2)  [unwired: 3 in, 2 out]
                              n137 = Equal?(x=w239, y=Error_Code_Enum_typedef."DRV_IDLE" ("status")) -> (x = y?=w238:bool)
                            }
                            frame #1 {
                              n138 = Wait (ms)(milliseconds to wait=u32 100) -> ()  [unwired: 1 out]
                            }
                          }
                        }
                      }
                      frame #2 {
                        n139 = Equal?(x=w245, y=u32 20002) -> (x = y?=w243:bool)
                        n140 = case shown="True" w243 {
                          tunnel: [i32[][] [] w247] -> w242
                          frame False {
                          }
                          frame True {
                            w248 = 512
                            n141 = To Long Integer(number=w248) -> (32bit integer=w250:i32)
                            n142 = To Long Integer(number=w248) -> (32bit integer=w249:i32)
                            n143 = Multiply(x=w250, y=w249) -> (x*y=w254:i32)
                            n144 = call <userlib>:"GetAcquiredData.vi"("size"=w254) -> ("DLL error code"=→"Return  from Get Acquired Data 2":u32, "array"=w252:i32[])  [unwired: 2 in, 1 out]
                            n145 = Multiply(x=1, y=w252) -> (x*y=w251:i32[])
                            n146 = Reshape Array(w251, w249, w250) -> (w247:i32[][])
                            n147 = local write "Intensity Graph 2"(w247) -> ()
                          }
                        }
                      }
                    }
                  }
                }
              }
              n148 = property on="Waveform Graph" class="WFGraph (strict)"("XScale.Multiplier"=w138, "XScale.Offset"=w137) -> ()  [unwired: 2 in, 2 out]
              n149 = property on="Intensity Graph 2" class="IntGraph (strict)"("XScale.Offset"=w137, "XScale.Multiplier"=w138) -> ()  [unwired: 2 in, 2 out]
              n150 = property on="Intensity Graph" class="IntGraph (strict)"("XScale.Multiplier"=w131) -> ()  [unwired: 2 in, 2 out]
              n151 = Initialize Array(0 ("element")) -> (w153:i32[][][])  [unwired: 3 in]
              n152 = for {
                N: 512 -> [_]
                tunnel: w158 -> [w215]
                shift-right: [w212] -> w147
                shift-left: w153 -> [w211]
                i -> [w210]
                n153 = Index Array(array=w215, index (dim 1)=w210) -> (element=w214:i32[][])  [unwired: 2 in]
                n154 = Transpose 2D Array(2D array=w214) -> (transposed array=w213:i32[][])
                n155 = Insert Into Array(array=w211, index (dim 1)=w210, new element=w213) -> (w212:i32[][][])  [unwired: 2 in]
              }
              n156 = Array Size(array=w158) -> (size(s)=→"size(s)":i32[])
              n157 = property on="total scan length(mm)" class="DigNum (strict)"() -> ("Value"=w152:dbl)  [unwired: 2 in, 2 out]
              n158 = local read "exposure time (s)"() -> (w136:sgl)
              n159 = Multiply(x=w152, y=1000) -> (x*y=w159:dbl)
              n160 = Array Size(array=w147) -> (size(s)=→"size(s) 2":i32[])
              n161 = Number To Decimal String(number=w159) -> (decimal integer string=w161:string)  [unwired: 1 in]
              n162 = Multiply(x=w136, y=sgl 1000.0) -> (x*y=w135:sgl)
              n163 = disable-structure shown="Enabled" {
                disable-tunnel: w147 -> [w204 w209]
                disable-tunnel: w135 -> [w203 _]
                disable-tunnel: w133 -> [w202 _]
                frame Enabled {
                  n164 = Path To String(path="Path") -> (string=w200:string)
                  n165 = Concatenate Strings(w200, "\\" ("string"), "File name", ".tiff" ("string")) -> (w197:string)
                  n166 = String To Path(string=w197) -> (path=w196:path)
                  n167 = call "saveToTIFF.vi"("x array"=w202, "Array"=w204, "selected path"=w196, "SPEC.CCD.Exposure(ms )"=w203) -> ()  [unwired: 7 in]
                  n168 = Index Array(array=w204, index (dim 0)=175 ("index (page)")) -> (element=w205:i32[][])  [unwired: 2 in]
                  n169 = local write "Intensity Graph"(w205) -> ()
                }
                frame Disabled {
                  n170 = Index Array(array=w209, index (dim 0)=175 ("index (page)")) -> (element=w207:i32[][])  [unwired: 2 in]
                  n171 = local write "Intensity Graph"(w207) -> ()
                }
              }
              n172 = disable-structure shown="Enabled" {
                disable-tunnel: w147 -> [w187 _]
                frame Enabled {
                  n173 = Open/Create/Replace File(file path (use dialog)="file path (use dialog)") -> (refnum out=w189:refnum<file>)  [unwired: 5 in, 2 out]
                  n174 = Write to Binary File(file (use dialog)=w189, data=w187, 9:T10."big-endian, network order" ("byte order (0:big-endian, network order)")) -> (refnum out=w188:refnum<file>)  [unwired: 3 in, 2 out]
                  n175 = Close File(refnum=w188) -> ()  [unwired: 1 in, 2 out]
                }
                frame Disabled {
                }
              }
              n176 = Concatenate Strings("a1#p" ("string"), w161, "dg" ("string"), "\r" ("write buffer")) -> (w160:string)
              n177 = VISA Write(VISA resource name=w168, write buffer=w160, error in (no error)=w167) -> (VISA resource name out=w165:refnum<visa-resource-name>, error out=w166:errorcluster)  [unwired: 1 out]
              n178 = VISA Close(VISA resource name=w165, error in (no error)=w166) -> (error out=w148:errorcluster)
            }
          }
          frame #2 {
            n179 = in-place {
              in-place-border: w265 -> [w268]
              in-place-border: [w267] -> w264
              in-place-border: [w266] -> w263
              n180 = while {
                tunnel: w268 -> [w282]
                tunnel: ["stop"] -> w267
                tunnel: ["scan again"] -> w266
                stop <- w271 stop-if-true
                n181 = event shown="[1] Timeout" {
                  selector: _ -> [_ _]
                  dyn-events: _ -> [_ _]
                  timeout: 10 -> [_ _]
                  tunnel: w282 -> [w363 _]
                  event "Intensity Graph": Mouse Down {
                    # "<-- asymmetry"
                    # "Needed because panel (0,0) is at TOP left rather than bottom left."
                    n182 = event-data() -> ("Coords"=w330:T11)  [unwired: 1 in, 2 out]
                    n183 = control-ref of="Intensity Graph"() -> (w324:refnum<vi>)
                    n184 = property on="Property Node" class="IntensityGraph (strict)"(reference=w324) -> ("X Scale.Range:Maximum"=w337:dbl, "X Scale.Range:Minimum"=w336:dbl, "Plot Area:Size:Width"=w335:u32, "Plot Area:Position:Left"=w334:i32)  [unwired: 1 in, 2 out]
                    n185 = property on="Property Node" class="IntensityGraph (strict)"(reference=w324) -> ("Y Scale.Range:Maximum"=w361:dbl, "Y Scale.Range:Minimum"=w356:dbl, "Plot Area:Size:Height"=w353:u32, "Plot Area:Position:Top"=w346:i32)  [unwired: 1 in, 2 out]
                    n186 = Unbundle By Name(w330) -> ("Horizontal"=w333:i32)
                    n187 = Unbundle By Name(w330) -> ("Vertical"=w360:i32)
                    n188 = To Double Precision Float(number=w333) -> (double precision float=w341:dbl)
                    n189 = To Double Precision Float(number=w346) -> (double precision float=w351:dbl)
                    n190 = To Double Precision Float(number=w360) -> (double precision float=w352:dbl)
                    n191 = To Double Precision Float(number=w334) -> (double precision float=w342:dbl)
                    n192 = To Double Precision Float(number=w335) -> (double precision float=w345:dbl)
                    n193 = To Double Precision Float(number=w353) -> (double precision float=w347:dbl)
                    n194 = Subtract(x=w341, y=w342) -> (x-y=w331:dbl)
                    n195 = Subtract(x=w352, y=w351) -> (x-y=w354:dbl)
                    n196 = Subtract(x=w347, y=w354) -> (x-y=w350:dbl)
                    n197 = In Range and Coerce(upper limit=w345, x=w331, lower limit=0.0) -> (coerced(x)=w344:dbl)  [unwired: 1 out]
                    n198 = In Range and Coerce(upper limit=w347, x=w350, lower limit=0.0) -> (coerced(x)=w348:dbl)  [unwired: 1 out]
                    n199 = Subtract(x=w337, y=w336) -> (x-y=w338:dbl)
                    n200 = Divide(x=w344, y=w345) -> (x/y=w339:dbl)
                    n201 = Subtract(x=w361, y=w356) -> (x-y=w359:dbl)
                    n202 = Divide(x=w348, y=w347) -> (x/y=w358:dbl)
                    n203 = Multiply(x=w338, y=w339) -> (x*y=w340:dbl)
                    n204 = Multiply(x=w359, y=w358) -> (x*y=w357:dbl)
                    n205 = Add(x=w340, y=w336) -> (x+y=w332:dbl)
                    n206 = Add(x=w357, y=w356) -> (x+y=w355:dbl)
                    n207 = Round To Nearest(number=w332) -> (nearest integer value=w325:dbl)
                    n208 = Round To Nearest(number=w355) -> (nearest integer value=w326:dbl)
                    n209 = Bundle(w325, w326) -> (w329:cluster{dbl, dbl})  [unwired: 1 in]
                    n210 = Unbundle(w329) -> (w328:dbl, w327:dbl)
                    n211 = Index Array(array=w363, index (dim 1)=w327, index (dim 2)=w328) -> (element=→"Waveform Graph":i32[])  [unwired: 1 in]
                  }
                  event Timeout {
                    n212 = event-data() -> ()  [unwired: 1 in, 3 out]
                  }
                }
                n213 = Array Size(array=w282) -> (size(s)=w284:i32[])
                n214 = Less?(x="Bandwidth", y="index (page) 2") -> (x < y?=w277:bool)
                n215 = Not Equal?(x="Bandwidth", y=0.0) -> (x != y?=w276:bool)
                n216 = Index Array(array=w284, index=2) -> (element=w281:i32)
                n217 = Index Array(array=w284, index=1) -> (element=w280:i32)
                n218 = And(x=w277, y=w276) -> (x .and. y?=w275:bool)
                n219 = Multiply(x=2.0, y="Bandwidth") -> (x*y=w286:dbl)
                n220 = Index Array(array=w282, index (dim 0)="index (page) 2") -> (element=w291:i32[][])  [unwired: 2 in]
                n221 = event shown="[1] \"Bandwidth\", \"index (page) 2\": Value Change" {
                  selector: _ -> [_ _]
                  dyn-events: _ -> [_ _]
                  timeout: 10 -> [_ _]
                  tunnel: [w293 w301] -> w290
                  tunnel: w291 -> [_ _]
                  tunnel: "index (page) 2" -> [_ w300]
                  tunnel: "Bandwidth" -> [_ w299]
                  tunnel: w282 -> [_ w298]
                  tunnel: w286 -> [_ w297]
                  tunnel: w281 -> [_ w296]
                  tunnel: w280 -> [_ w295]
                  tunnel: w275 -> [_ w294]
                  event Timeout {
                    n222 = event-data() -> ()  [unwired: 1 in, 3 out]
                    n223 = local read "Intensity Graph"() -> (w293:i32[][])
                  }
                  event "Bandwidth", "index (page) 2": Value Change {
                    n224 = event-data() -> ()  [unwired: 1 in, 6 out]
                    n225 = case shown="True" w294 {
                      tunnel: w300 -> [w304 w313]
                      tunnel: w298 -> [w303 w314]
                      tunnel: w297 -> [_ w305]
                      tunnel: [w302 w312] -> w301
                      tunnel: w299 -> [_ w311]
                      tunnel: w296 -> [_ w308]
                      tunnel: w295 -> [_ w307]
                      frame False {
                        n226 = Index Array(array=w303, index (dim 0)=w304) -> (element=w302:i32[][])  [unwired: 2 in]
                      }
                      frame True {
                        n227 = Initialize Array(0 ("element"), w307, w308) -> (w309:i32[][])
                        n228 = for {
                          N: w305 -> [_]
                          tunnel: w314 -> [w323]
                          shift-right: [w321] -> w306
                          shift-left: w309 -> [w318]
                          tunnel: w313 -> [w317]
                          tunnel: w311 -> [w316]
                          i -> [w322]
                          n229 = Subtract(x=w317, y=w316) -> (x-y=w315:dbl)
                          n230 = Add(x=w322, y=w315) -> (x+y=w320:dbl)
                          n231 = Index Array(array=w323, index (dim 0)=w320) -> (element=w319:i32[][])  [unwired: 2 in]
                          n232 = Add ("Add.vi")(x=w319, y=w318) -> (x+y=w321:i32[][])
                        }
                        n233 = Divide(x=w306, y=w305) -> (x/y=w312:dbl[][])
                      }
                    }
                  }
                }
                n234 = Divide(x="Y Scale Range (mm)", y=512.0) -> (x/y=w274:dbl)
                n235 = property on="Intensity Graph 2" class="IntGraph (strict)"("YScale.Multiplier"=w274) -> ()  [unwired: 2 in, 2 out]
                n236 = property on="Intensity Graph" class="IntGraph (strict)"("YScale.Multiplier"=w274) -> ()  [unwired: 2 in, 2 out]
                n237 = local write "Intensity Graph"(w290) -> ()
                n238 = Or(x="scan again", y="stop") -> (x .or. y?=w271:bool)
              }
            }
          }
          frame #3 {
            n239 = case shown="True" w364 {
              frame False {
              }
              frame True {
                n240 = property on="Tab Control" class="TabCtl (strict)"("Value"=T1."Acquire" ("Tab Control")) -> ()  [unwired: 2 in, 2 out]
              }
            }
            n241 = Wait (ms)(milliseconds to wait=u32 1000) -> ()  [unwired: 1 out]
          }
        }
      }
    }
    frame #2 {
      n242 = flat-sequence {
        frame #0 {
          n243 = in-place {
            n244 = call <userlib>:"CoolerOFF.vi"() -> ("error out"=w367:errorcluster)  [unwired: 2 in, 1 out]
            n245 = call <userlib>:"SetShutter.vi"("type"=Shutter_type_typedef."TTL Low", "mode"=Shutter_mode_typedef."Close", "error in (no error)"=w367) -> ()  [unwired: 11 in, 2 out]
            n246 = while {
              stop <- w371 stop-if-true
              n247 = flat-sequence {
                tunnel: [w374] -> w371
                frame #0 {
                  n248 = call <userlib>:"GetTemperature.vi"() -> ("status"=w372:T2, "temperature"=w373:i32)  [unwired: 4 in, 2 out]
                  n249 = local write "temperature 2"(w373) -> ()
                  n250 = local write "temp. status 2"(w372) -> ()
                  n251 = Greater Or Equal?(x=w373, y=0) -> (x >= y?=w374:bool)
                }
                frame #1 {
                  n252 = Wait (ms)(milliseconds to wait=u32 2000) -> ()  [unwired: 1 out]
                }
              }
              n253 = Not(x=w371) -> (.not. x?=→"recovering temperature":bool)
            }
          }
        }
        frame #1 {
          n254 = in-place {
            n255 = call <userlib>:"AbortAcquisition.vi"() -> ("error out"=w377:errorcluster)  [unwired: 2 in, 1 out]
            n256 = call <userlib>:"ShutDown.vi"("error in (no error)"=w377) -> ()  [unwired: 1 in, 2 out]
          }
        }
      }
    }
  }
